vi "New Control Caption Binding.vi"(10 "Ctl Refnum":refnum<vi>) -> (0 "error out":errorcluster, 3 "ControlCaptionBinding":refnum<class "ControlCaptionBinding.lvclass">)   [LabVIEW 2017, in "Transport.lvlib" / "ControlCaptionBinding.lvclass"]
doc: "<License>\nCopyright © 2017 Composed Systems, LLC | All rights reserved\nwww.composed.io\n\nAuthor: Ethan Stern <ethan.stern@composed.io>\n\nThis software is provided \"AS IS\" WITHOUT WARRANTIES, either express or implied, AND IS FOR EDUCATIONAL PURPOSES ONLY.\n</License>"
uses:
  ControlCaptionBinding.lvclass
  ControlCaptionBinding.lvclass/ControlCaptionBinding.ctl
  <vilib>/Utility/error.llb/Error Cluster From Error Code.vi
  <vilib>/ErrorRing/Error Ring.xnode
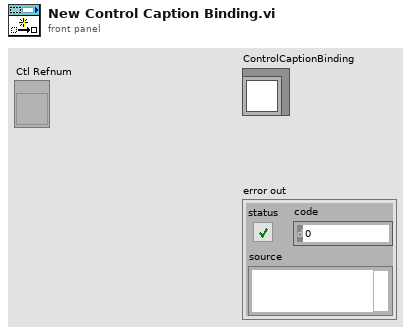
[diagram p1: front panel]
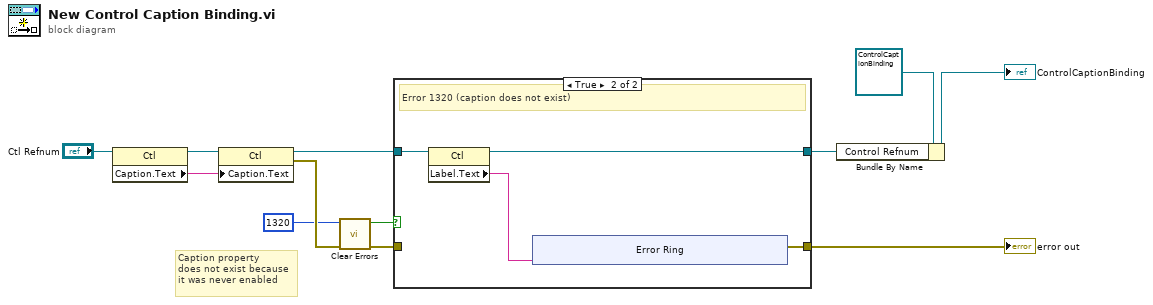
[diagram p0: block diagram]
diagram:
  # "Caption property\ndoes not exist because\nit was never enabled"
  n1 = property class="Ctl"(reference="Ctl Refnum") -> (reference out=w2:refnum<vi>, "Caption.Text"=w1:string)  [unwired: 1 in, 1 out]
  n2 = property class="Ctl"(reference=w2, "Caption.Text"=w1) -> (reference out=w8:refnum<vi>, error out=w5:errorcluster)  [unwired: 1 in]
  n3 = call <vilib>:"Clear Errors.vi"("error in (no error)"=w5, "specific error code to clear (0: all)"=1320) -> ("error out"=w4:errorcluster, "specific error cleared?"=w6:bool)  [unwired: 4 in]
  n4 = case shown="True" w6 {
    tunnel: [w13 w18] -> w9
    tunnel: w8 -> [w14 w17]
    tunnel: [w14 w16] -> w7
    tunnel: w4 -> [w13 _]
    frame False {
    }
    frame True {
      # "Error 1320 (caption does not exist)"
      n5 = property class="Ctl"(reference=w17) -> (reference out=w16:refnum<vi>, "Label.Text"=w15:string)  [unwired: 1 in, 1 out]
      n6 = xnode "Error Ring"("parameter 0"=w15) -> ("error out"=w18:errorcluster)
    }
  }
  "error out" <- w9
  n7 = Bundle By Name(cluster=refnum<class "ControlCaptionBinding.lvclass"> refnum ("TerminalBinding in"), "Control Refnum"=w7) -> (→"ControlCaptionBinding":refnum<class "ControlCaptionBinding.lvclass">)
